vi "Emballage_BDD_messageRemplaceValve.vi"(8 "Error in":errorcluster caption="Error in (no error)", 10 "SN_RPODUIT_ancien":string, 11 "SN_PRODUIT remplacant":string) -> (0 "Error out":errorcluster, 3 "btn_Continuer 2":bool)   [LabVIEW 2020]
uses:
  Modules/FS/60_FS_Controles/60_FS_SetGet.ctl
panel:
  in  "btn_Continuer":bool
  in  "Bouton Annuler":bool
  out "Message":string
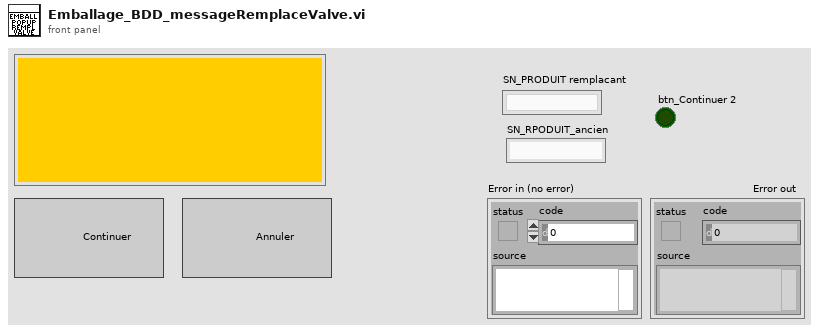
[diagram p1: front panel]
types:
  T1 = typedef "60_FS_SetGet.ctl" = enum16{"set", "get"}
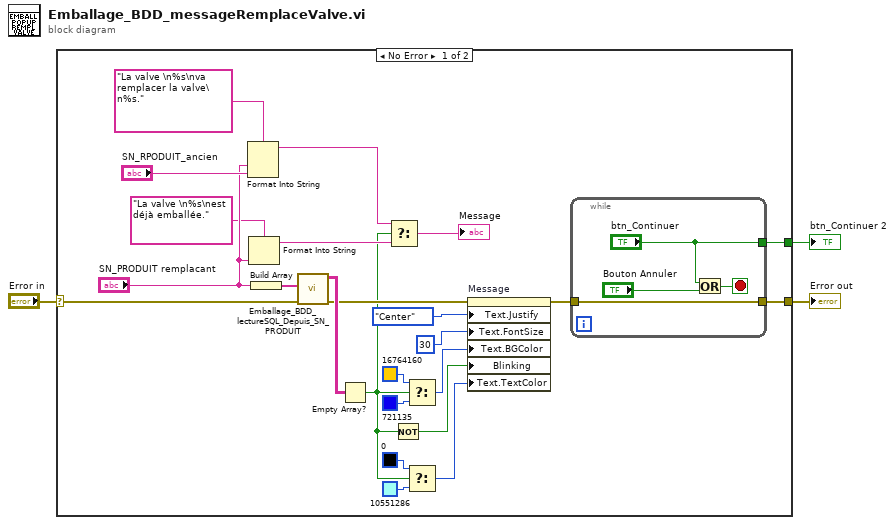
[diagram p0: block diagram]
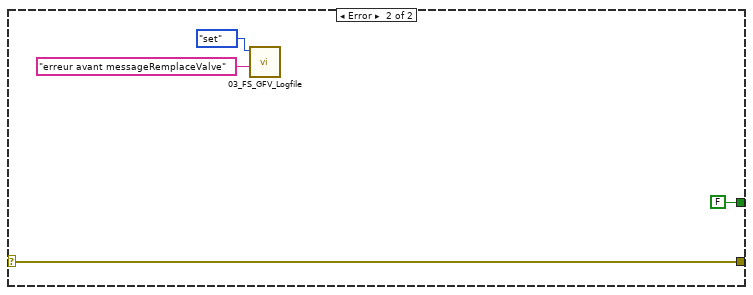
[diagram p2: hidden frame]
diagram:
  n1 = case shown="No Error" "Error in" {
    selector: "Error in" -> [w7 w35]
    tunnel: [w6 w35] -> w2
    tunnel: [w5 FALSE ("btn_Continuer")] -> w1
    frame No Error {
      n2 = Format Into String(format string="La valve \n%s\nva remplacer la valve\n%s." ("Message"), "SN_PRODUIT remplacant", "SN_RPODUIT_ancien") -> (resulting string=w25:string)  [unwired: 2 in, 1 out]
      n3 = Format Into String(format string="La valve \n%s\nest déjà emballée." ("Message"), "SN_PRODUIT remplacant") -> (resulting string=w22:string)  [unwired: 2 in, 1 out]
      n4 = Build Array("SN_PRODUIT remplacant") -> (w4:string[])
      n5 = call "Emballage_BDD_lectureSQL_Depuis_SN_PRODUIT.vi"("Error in"=w7, "Where (Valeur)"=w4) -> ("Error out"=w19:errorcluster, "Donnees"=w27:string[][])  [unwired: 7 in, 1 out]
      n6 = Empty Array?(array=w27) -> (empty?=w10:bool)
      n7 = Select(t=w25, s=w10, f=w22) -> (s? t:f=→"Message":string)
      n8 = Not(x=w10) -> (.not. x?=w14:bool)
      n9 = Select(t=u32 16764160, s=w10, f=u32 721135) -> (s? t:f=w15:u32)
      n10 = Select(t=u32 0, s=w10, f=u32 10551286) -> (s? t:f=w12:u32)
      n11 = property on="Message" class="Str"(error in=w19, "Text.Justify"=enum16{"Left", "Center", "Right"}."Center" ("Texte.Justification"), "Text.FontSize"=u32 30 ("Texte.Police:Taille"), "Text.BGColor"=w15, "Blinking"=w14, "Text.TextColor"=w12) -> (error out=w13:errorcluster)  [unwired: 1 in, 1 out]
      n12 = while {
        tunnel: [w31] -> w6
        tunnel: w13 -> [w31]
        tunnel: ["btn_Continuer"] -> w5
        stop <- w30 stop-if-true
        n13 = Or(x="btn_Continuer", y="Bouton Annuler") -> (x .or. y?=w30:bool)
      }
    }
    frame Error {
      n14 = call "03_FS_GFV_Logfile.vi"("Chaîne"="erreur avant messageRemplaceValve", "States"=60_FS_SetGet."set") -> ()  [unwired: 8 in, 2 out]
    }
  }
  "Error out" <- w2
  "btn_Continuer 2" <- w1
